vi "CleanUp.vi"(8 "error in (no error)":errorcluster, 11 "object in":refnum<class "Type-T-Thermocouple.lvclass">) -> (0 "error out":errorcluster, 3 "object out":refnum<class "Type-T-Thermocouple.lvclass">)   [LabVIEW 2016, in "Type-T-Thermocouple.lvclass"]
uses:
  Type-T-Thermocouple.lvclass
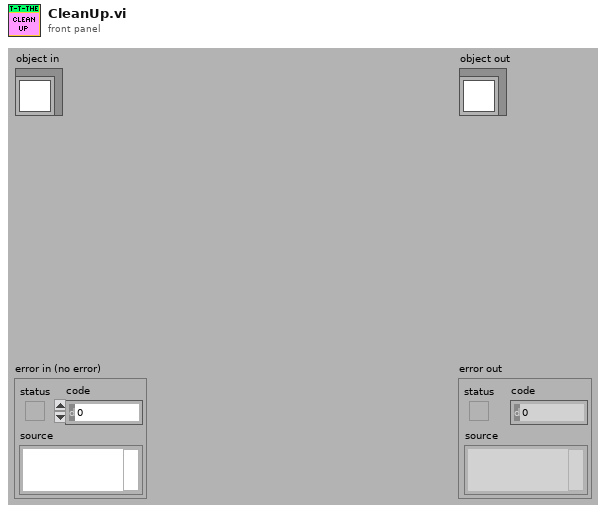
[diagram p1: front panel]
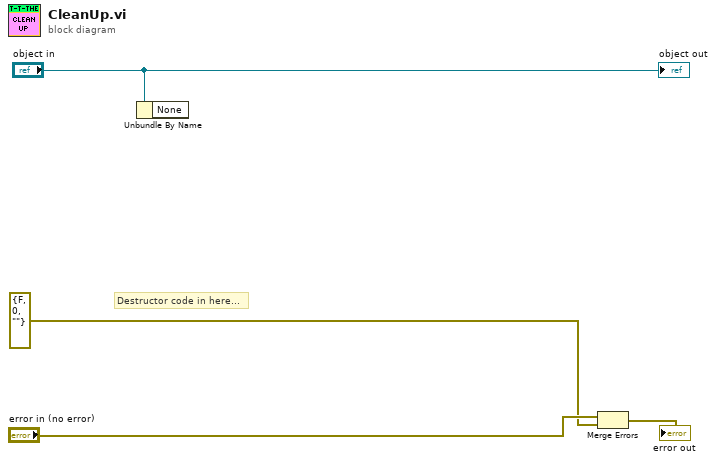
[diagram p0: block diagram]
diagram:
  # "Destructor code in here..."
  n1 = Unbundle By Name("object in") -> ()  [unwired: 1 out]
  n2 = Merge Errors("error in (no error)", errorcluster {"status"=FALSE, "code"=0, "source"=""} ("error in (no error)")) -> (→"error out":errorcluster)
  "object out" <- "object in"
